vi "SubVI_InitialUI_ResetPanes.vi"   [LabVIEW 2011]
uses:
  <vilib>/Utility/miscctls.llb/LVPointTypeDef.ctl
types:
  T1 = typedef "LVPointTypeDef.ctl" = cluster{"Horizontal":i16, "Vertical":i16}
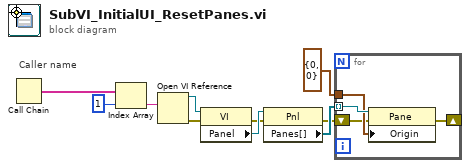
[diagram p0: block diagram]
diagram:
  # "Caller name"
  n1 = Call Chain() -> (call chain=w6:string[])
  n2 = Index Array(array=w6, index=1) -> (element=w7:string)
  n3 = Open VI Reference(vi path=w7) -> (vi reference=w4:refnum<vi>, error out=w3:errorcluster)  [unwired: 5 in]
  n4 = property class="VI"(reference=w4, error in=w3) -> (error out=w2:errorcluster, "Panel"=w8:refnum<vi>)  [unwired: 1 out]
  n5 = property class="Pnl"(reference=w8, error in=w2) -> (error out=w1:errorcluster, "Panes[]"=w9:refnum<vi>[])  [unwired: 1 out]
  n6 = for {
    tunnel: w9 -> [w14] mode=indexing
    tunnel: T1 {"Horizontal"=0, "Vertical"=0} ("Origin") -> [w13]
    shift-right: [w11] -> _
    shift-left: w1 -> [w12]
    n7 = property on="Property Node" class="Pane"(reference=w14, error in=w12, "Origin"=w13) -> (error out=w11:errorcluster)  [unwired: 1 out]
  }
